vi "Read Environment Variable.vi"(8 "error in":errorcluster, 11 "name":string="NIDATASTORE_DATASTORESETTINGS__FAILEDINGESTDIRECTORY") -> (0 "error out":errorcluster, 3 "value":string)   [LabVIEW 2024]
uses:
  <vilib>/Utility/error.llb/Trim Whitespace One-Sided.vi
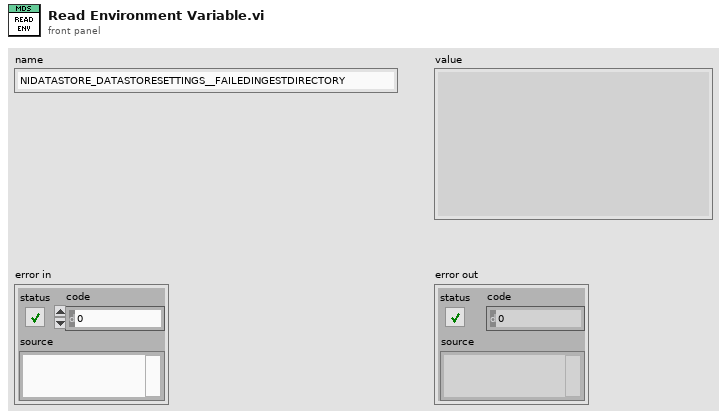
[diagram p1: front panel]
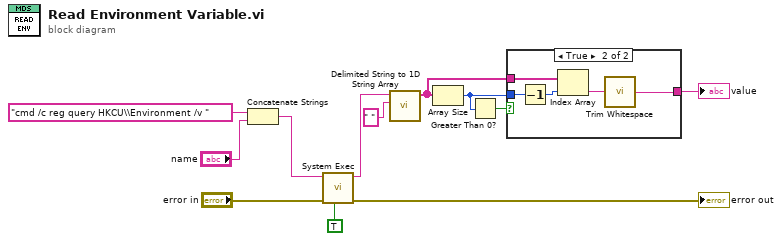
[diagram p0: block diagram]
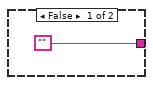
[diagram p2: hidden frame]
diagram:
  n1 = Concatenate Strings("cmd /c reg query HKCU\\Environment /v " ("string"), "name") -> (w8:string)
  n2 = call <vilib>:"System Exec.vi"("run minimized? (F)"=TRUE, "error in (no error)"="error in", "command line"=w8) -> ("error out"=→"error out":errorcluster, "standard output"=w1:string)  [unwired: 5 in, 2 out]
  n3 = call <vilib>:"Delimited String to 1D String Array.vi"("delimiter"=" ", "delimited string"=w1) -> ("string array"=w6:string[])  [unwired: 9 in]
  n4 = Array Size(array=w6) -> (size(s)=w4:i32)
  n5 = Greater Than 0?(x=w4) -> (x > 0?=w3:bool)
  n6 = case shown="True" w3 {
    tunnel: w4 -> [_ w18]
    tunnel: w6 -> [_ w16]
    tunnel: ["" w14] -> w5
    frame False {
    }
    frame True {
      n7 = Decrement(x=w18) -> (x-1=w17:i32)
      n8 = Index Array(array=w16, index=w17) -> (element=w15:string)
      n9 = call <vilib>:"Trim Whitespace.vi"("string"=w15) -> ("trimmed string"=w14:string)  [unwired: 1 in]
    }
  }
  "value" <- w5
